vi "OutToFileConfig.vi"(8 "error in (no error)":errorcluster, 11 "OutputToFileBasePlugin in":refnum<class "OutputToFileBasePlugin.lvclass">) -> (0 "error out":errorcluster, 3 "OutputToFileBasePlugin out":refnum<class "OutputToFileBasePlugin.lvclass">)   [LabVIEW 2017, in "OutputToFilePlugins.lvlib" / "OutputToFileBasePlugin.lvclass"]
uses:
  OutputToFileBasePlugin.lvclass
  Typedefs/PmuCfgOpt.ctl
  OutputToFileBasePlugin.lvclass/OutputToFileBasePlugin.ctl
  Framework/Config_class/Config.lvclass/Config.ctl
  Accessors/Write clConfigOptions.vi
  Accessors/Write OutputPath.vi
  Framework/Config_class/Accessors/Write PARTF Root Directory.vi
  Framework/Config_class/Accessors/Read PARTF Root Directory.vi
  Accessors/Read clConfigOptions.vi
  Framework/Config_class/Config.lvclass
  <vilib>/Utility/config.llb/NI_LVConfig.lvlib
panel:
  in  "BtnCancel":bool
  in  "btnSave":bool
  in  "btnOutPath":bool
  out "Output File Path":path caption="To change the root data directory use the \"Settings\" button"
  in  "clConfigOptions":T1={"TIME_BASE"=1000000, "STN"="Bus_1", "IDCODE"=0, "rdoPolRect"=enum."Rectangular", "rdoFloatInt"=enum."Float", "PHUNIT"=1000000, "rdoFreqDfreq"=enum."Float", "CHNAM"=["VA", "VB", "VC", "V+", "IA", "IB", "IC", "I+"], "chkCfg2Prefix"=TRUE} caption="PMU Configuration Options" {"PHUNIT" max=16777216 step=1 format="%08d"; "IDCODE" format="%02x"; "TIME_BASE" max=16777216 step=1 format="%08d"}
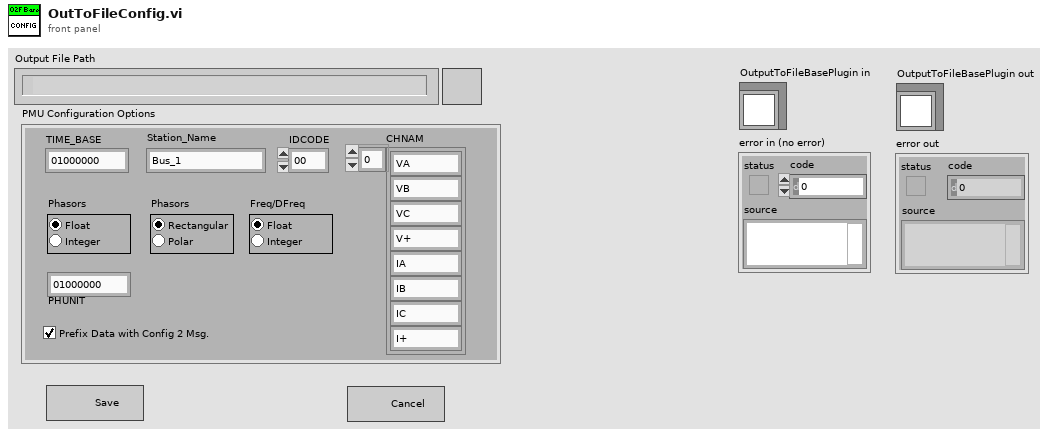
[diagram p1: front panel]
types:
  T1 = typedef "OutputToFilePlugins.lvlib/OutputToFileBasePlugin.lvclass/PmuCfgOpt.ctl" = cluster{"TIME_BASE":u64, "STN":string, "IDCODE":u16, "rdoPolRect":enum32{"Rectangular", "Polar"}, "rdoFloatInt":enum32{"Float", "Integer"}, "PHUNIT":u64, "rdoFreqDfreq":enum32{"Float", "Integer"}, "CHNAM":string[], "chkCfg2Prefix":bool}
  T2 = typedef "Framework.lvlib/Config.lvclass/RootDir.ctl" = cluster{"pathRootDir":path, "btnOutPath":bool, "OutDir":string, "btnOpenOutputDir":bool, "ScriptDir":string, "btnOpenScriptDir":bool, "TestDir":string, "btnOpenTestDir":bool}
  T3 = typedef "NI_LVConfig.lvlib/Config Data RefNum.ctl" = refnum<k1>
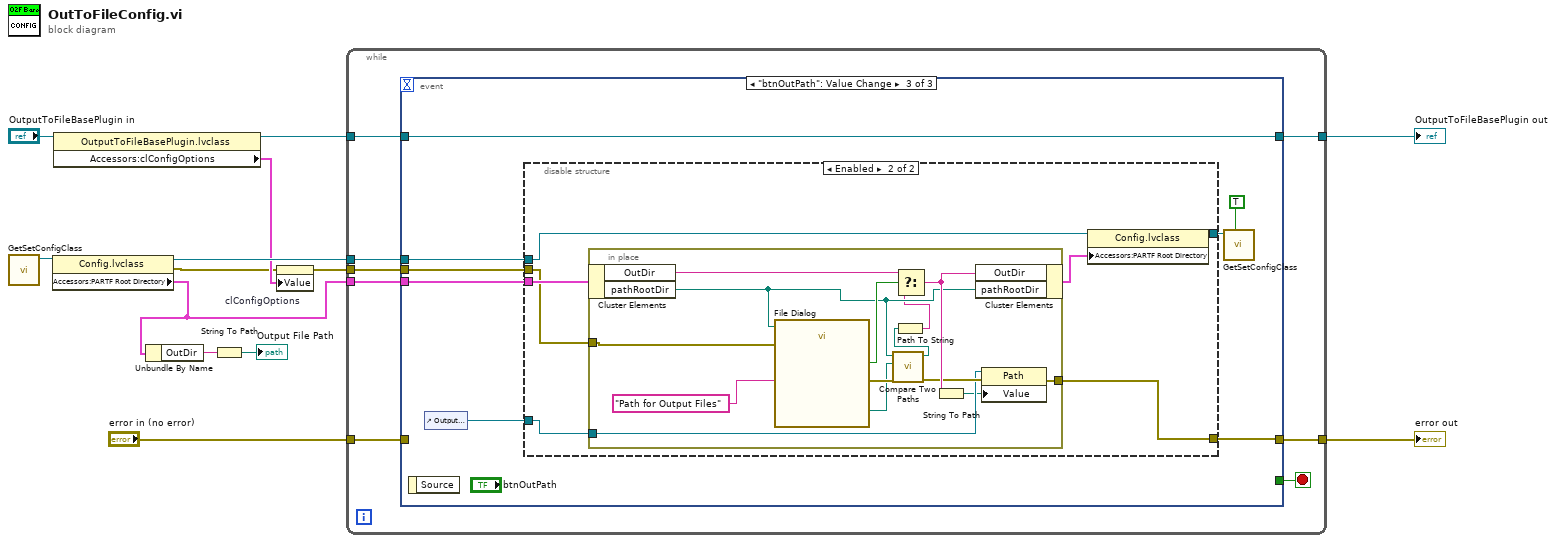
[diagram p0: block diagram]
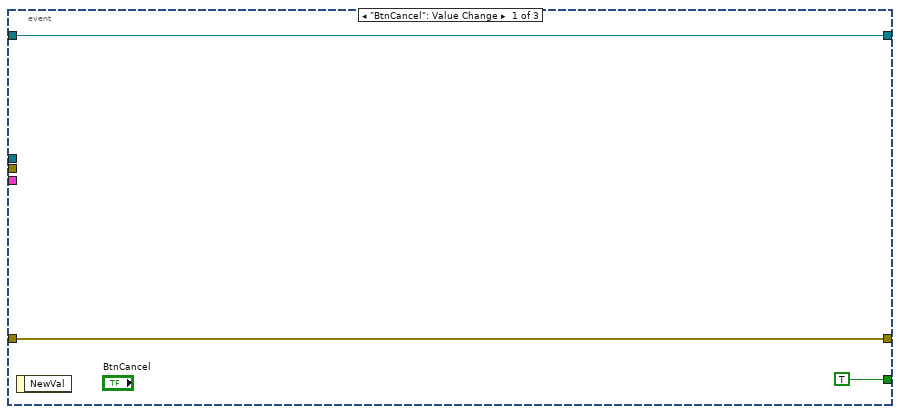
[diagram p2: hidden frame]
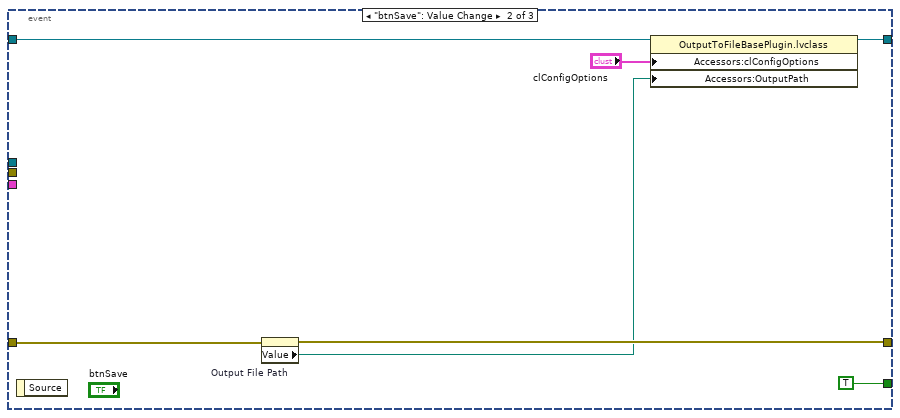
[diagram p3: hidden frame]
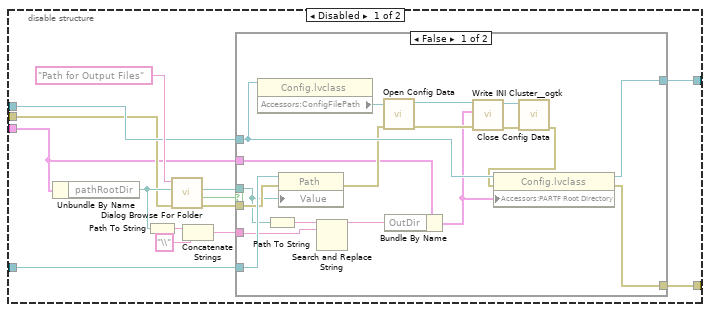
[diagram p4: hidden frame]
diagram:
  n1 = call "GetSetConfigClass.vi"() -> ("Ref out"=w10:refnum<class "Config.lvclass">)  [unwired: 11 in]
  n2 = property class="Config.lvclass"(reference=w10) -> (reference out=w7:refnum<class "Config.lvclass">, error out=w3:errorcluster, "Accessors:PARTF Root Directory"=w4:T2)  [unwired: 1 in]
  n3 = property class="OutputToFileBasePlugin.lvclass"(reference="OutputToFileBasePlugin in") -> (reference out=w1:refnum<class "OutputToFileBasePlugin.lvclass">, "Accessors:clConfigOptions"=w5:T1)  [unwired: 1 in, 1 out]
  n4 = Unbundle By Name(w4) -> ("OutDir"=w9:string)
  n5 = String To Path(string=w9) -> (path=→"Output File Path":path)
  n6 = property on="clConfigOptions" class="Clust (strict)"(error in=w3, "Value"=w5) -> (error out=w2:errorcluster)  [unwired: 1 in, 1 out]
  n7 = while {
    tunnel: w1 -> [w21]
    tunnel: "error in (no error)" -> [w19]
    tunnel: [w20] -> w12
    tunnel: [w18] -> w11
    tunnel: w7 -> [w16]
    tunnel: w2 -> [w15]
    tunnel: w4 -> [w14]
    stop <- w17 stop-if-true
    n8 = event shown="[2] \"btnOutPath\": Value Change" {
      selector: _ -> [_ _ _]
      dyn-events: _ -> [_ _ _]
      timeout: _ -> [_ _ _]
      tunnel: w21 -> [w24 w30 w37]
      tunnel: [w24 w29 w37] -> w20
      tunnel: w19 -> [w23 w27 _]
      tunnel: [w23 w26 w38] -> w18
      tunnel: [TRUE TRUE _] -> w17
      tunnel: w16 -> [_ _ w36]
      tunnel: w15 -> [_ _ w35]
      tunnel: w14 -> [_ _ w34]
      event "BtnCancel": Value Change {
        n9 = event-data() -> ()  [unwired: 1 in, 1 out]
      }
      event "btnSave": Value Change {
        n10 = event-data() -> ()  [unwired: 1 in, 1 out]
        n11 = property on="Output File Path" class="Path"(error in=w27) -> (error out=w26:errorcluster, "Value"=w25:path)  [unwired: 1 in, 1 out]
        n12 = property class="OutputToFileBasePlugin.lvclass"(reference=w30, "Accessors:clConfigOptions"="clConfigOptions", "Accessors:OutputPath"=w25) -> (reference out=w29:refnum<class "OutputToFileBasePlugin.lvclass">)  [unwired: 1 in, 1 out]
      }
      event "btnOutPath": Value Change {
        n13 = event-data() -> ()  [unwired: 1 in, 1 out]
        n14 = control-ref of="Output File Path"() -> (w39:refnum<vi>)
        n15 = disable-structure shown="Enabled" {
          disable-tunnel: w39 -> [w45 w77]
          disable-tunnel: [w44 w76] -> w38
          disable-tunnel: w36 -> [w43 w75]
          disable-tunnel: w35 -> [w42 w78]
          disable-tunnel: w34 -> [w41 w79]
          disable-tunnel: [w40 w73] -> w33
          frame Disabled {
            n16 = Unbundle By Name(w41) -> ("pathRootDir"=w47:path)
            n17 = Path To String(path=w47) -> (string=w52:string)
            n18 = call "Dialog Browse For Folder.vi"("error in"=w42, "Root directory"=w47, "Title"="Path for Output Files") -> ("error out"=w48:errorcluster, "cancelled"=w49:bool, "Selected Path"=w50:path)  [unwired: 6 in]
            n19 = Concatenate Strings(w52, "\\" ("string")) -> (w46:string)
            n20 = case shown="False" w49 {
              tunnel: w45 -> [w71 _]
              tunnel: w50 -> [w69 _]
              tunnel: w48 -> [w70 _]
              tunnel: w43 -> [w65 w72]
              tunnel: [w56 _] -> w44
              tunnel: w46 -> [w66 _]
              tunnel: w41 -> [w55 _]
              tunnel: [w54 w72] -> w40
              frame False {
                n21 = property class="Config.lvclass"(reference=w65) -> ("Accessors:ConfigFilePath"=w64:path)  [unwired: 1 in, 2 out]
                n22 = Path To String(path=w69) -> (string=w68:string)
                n23 = property class="Path"(reference=w71, error in=w70, "Value"=w69) -> (error out=w61:errorcluster)  [unwired: 1 out]
                n24 = Search and Replace String(input string=w68, search string=w66) -> (result string=w67:string)  [unwired: 6 in, 3 out]
                n25 = call <vilib>:"Open Config Data.vi"("error in (no error)"=w61, "configuration file path"=w64) -> ("error out"=w63:errorcluster, "refnum"=w62:T3)  [unwired: 7 in, 1 out]
                n26 = Bundle By Name(cluster=w55, "OutDir"=w67) -> (w57:T2)
                n27 = call <userlib>:"Write INI Cluster__ogtk.vi"("error in (no error)"=w63, "INI Fomatted Cluster"=w57, "refnum"=w62) -> ("error out"=w60:errorcluster, "dup refnum"=w59:T3)  [unwired: 7 in]
                n28 = call <vilib>:"Close Config Data.vi"("error in (no error)"=w60, "refnum"=w59) -> ("error out"=w58:errorcluster)  [unwired: 8 in, 1 out]
                n29 = property class="Config.lvclass"(reference=w65, error in=w58, "Accessors:PARTF Root Directory"=w57) -> (reference out=w54:refnum<class "Config.lvclass">, error out=w56:errorcluster)
              }
              frame True {
              }
            }
          }
          frame Enabled {
            n30 = in-place {
              in-place-border: [w89] -> w76
              in-place-border: w78 -> [w93]
              in-place-border: w77 -> [w82]
              n31 = in-place-cluster #1(w79) -> ("OutDir"=w91:string, "pathRootDir"=w86:path)
              n32 = call "File Dialog"("start path"=w86, "prompt"="Path for Output Files" ("Title"), "error in"=w93) -> ("selected path"=w85:path, "cancelled"=w92:bool, "error out"=w88:errorcluster)  [unwired: 9 in, 1 out]
              n33 = call <vilib>:"Compare Two Paths.vi"("error in (no error)"=w88, "Path 2"=w85, "Path 1"=w86) -> ("error out"=w87:errorcluster, "Relative Path from 1 to 2"=w84:path)  [unwired: 5 in, 2 out]
              n34 = Path To String(path=w84) -> (string=w83:string)
              n35 = Select(t=w91, s=w92, f=w83) -> (s? t:f=w90:string)
              n36 = String To Path(string=w90) -> (path=w81:path)
              n37 = in-place-cluster #1("OutDir"=w90, "pathRootDir"=w86) -> (w74:T2)
              n38 = property on="Property Node" class="Path"(reference=w82, error in=w87, "Value"=w81) -> (error out=w89:errorcluster)  [unwired: 1 out]
            }
            n39 = property class="Config.lvclass"(reference=w75, "Accessors:PARTF Root Directory"=w74) -> (reference out=w73:refnum<class "Config.lvclass">)  [unwired: 1 in, 1 out]
          }
        }
        n40 = call "GetSetConfigClass.vi"("Set (f)"=TRUE, "Ref in"=w33) -> ()  [unwired: 9 in, 1 out]
      }
    }
  }
  "error out" <- w11
  "OutputToFileBasePlugin out" <- w12
